vi "MagX Start OSF Sync.vi"(8 "error in":errorcluster, 9 "Station":string="Cell_3", 10 "Experiment ID":string, 11 "MagLab OSF tool server":string="magx.lanl.gov") -> (0 "error out":errorcluster)   [LabVIEW 2020]
uses:
  3c8e3627-593a-4182-af88-7bff6491b42d.vi
  <vilib>/JDP Science/JSONtext/JSON text to Variant.vi
  <vilib>/JDP Science/JSONtext/LVClass Serializer/JSONtext LVClass Serializer.lvclass
  <vilib>/httpClient/LabVIEWHTTPClient.lvlib
panel:
  out "after substring":string
  out "headers":string
  out "body":string
  out "Data out":cluster{"user":string}
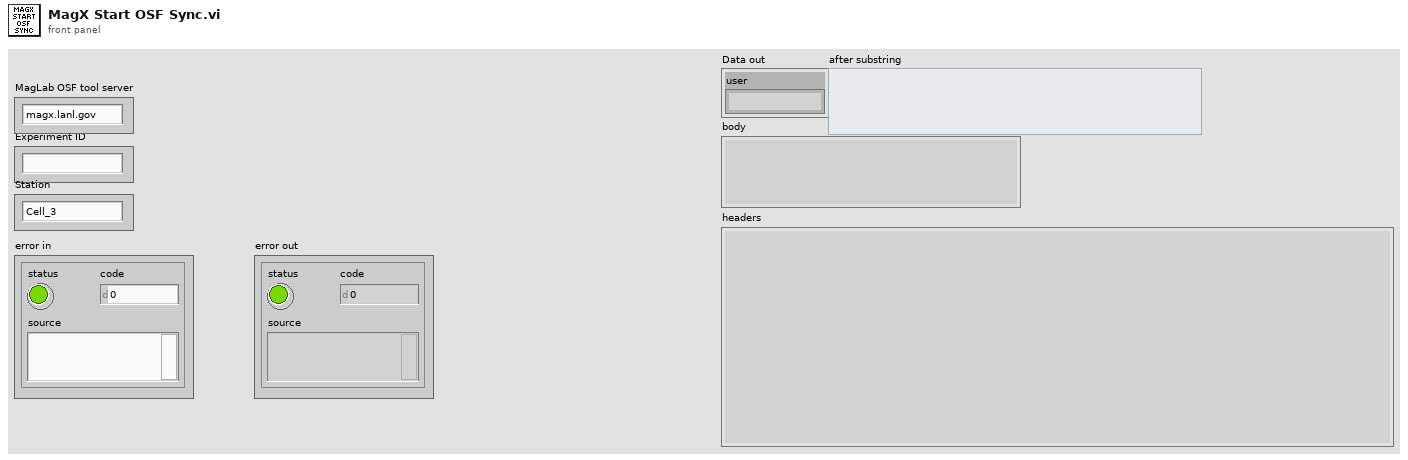
[diagram p1: front panel]
types:
  T1 = typedef "LabVIEWHTTPClient.lvlib/ClientHandle.ctl" = refnum<k1>
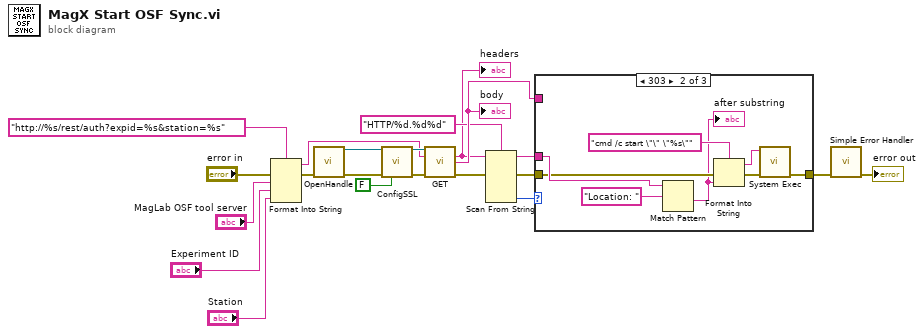
[diagram p0: block diagram]
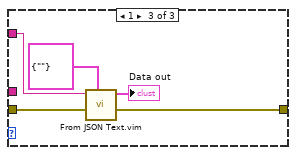
[diagram p3: hidden frame]
diagram:
  n1 = Format Into String(format string="http://%s/rest/auth?expid=%s&station=%s", error in="error in", "MagLab OSF tool server", "Experiment ID", "Station") -> (resulting string=w9:string, error out=w15:errorcluster)  [unwired: 1 in]
  n2 = call <vilib>:"OpenHandle.vi"("error in (no error)"=w15) -> ("client handle out"=w18:T1, "error out"=w19:errorcluster)  [unwired: 13 in]
  n3 = call <vilib>:"ConfigSSL.vi"("client handle"=w18, "error in (no error)"=w19, "verify server (true)"=FALSE) -> ("client handle out"=w21:T1, "error out"=w20:errorcluster)  [unwired: 11 in]
  n4 = call <vilib>:"GET.vi"("client handle"=w21, "url"=w9, "error in (no error)"=w20) -> ("headers"=w1:string, "body"=w17:string, "error out"=w6:errorcluster)  [unwired: 9 in, 1 out]
  "body" <- w17
  "headers" <- w1
  n5 = Scan From String(format string="HTTP/%d.%d%d", input string=w1, error in=w6) -> (remaining string=w2:string, error out=w3:errorcluster, output 3=w4:i32)  [unwired: 6 in, 1 out]
  n6 = case shown="303" w4 {
    tunnel: w17 -> [_ _ w35]
    tunnel: w3 -> [w22 w25 w34]
    tunnel: [w22 w24 w31] -> w13
    tunnel: w2 -> [_ w30 _]
    frame 0, Default {
    }
    frame 303 {
      n7 = Match Pattern(string=w30, regular expression="Location: ") -> (after substring=w23:string)  [unwired: 1 in, 3 out]
      "after substring" <- w23
      n8 = Format Into String(format string="cmd /c start \"\" \"%s\"" ("command line"), error in=w25, w23) -> (resulting string=w26:string, error out=w28:errorcluster)  [unwired: 1 in]
      n9 = call <vilib>:"System Exec.vi"("error in (no error)"=w28, "command line"=w26) -> ("error out"=w24:errorcluster)  [unwired: 6 in, 3 out]
    }
    frame 1 {
      n10 = call "From JSON Text.vim"("Data Type and Default Value"=cluster{"user":string} {"user"=""}, "error in (no error)"=w34, "JSON"=w35) -> ("error out"=w31:errorcluster, "Data out"=→"Data out":cluster{"user":string})  [unwired: 7 in]
    }
  }
  n11 = call <vilib>:"Simple Error Handler.vi"("error in (no error)"=w13) -> ("error out"=→"error out":errorcluster)  [unwired: 4 in, 4 out]
